vi "Setscope.vi"(10 "Set_Val":T1) -> (3 "OneOfTemplate out":refnum<class "nixnet_grpc_StartRequest_scope_enum.lvclass">)   [LabVIEW 2019, in "xnet-grpc_client.lvlib" / "nixnet_grpc_StartRequest_scope_enum.lvclass"]
uses:
  nixnet_grpc_StartRequest_scope_enum.lvclass
  nixnet_grpc_StartRequest_scope_enum.lvclass/nixnet_grpc_StartRequest_scope_enum.ctl
  nixnet_grpc_StartStopScope.ctl
  xnet-grpc_client.lvlib
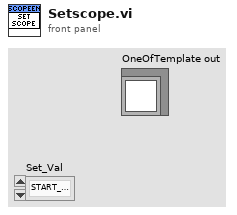
[diagram p1: front panel]
types:
  T1 = typedef "xnet-grpc_client.lvlib/nixnet_grpc_StartStopScope.ctl" = enum32{"START_STOP_SCOPE_NORMAL", "START_STOP_SCOPE_SESSION_ONLY", "START_STOP_SCOPE_INTERFACE_ONLY", "START_STOP_SCOPE_SESSION_ONLY_BLOCKING"}
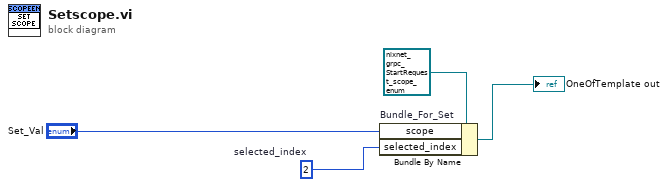
[diagram p0: block diagram]
diagram:
  w2 = 2  # selected_index
  n1 = Bundle By Name "Bundle_For_Set"(cluster=refnum<class "nixnet_grpc_StartRequest_scope_enum.lvclass"> refnum ("OneOfTemplate in"), "scope"="Set_Val", "selected_index"=w2) -> (→"OneOfTemplate out":refnum<class "nixnet_grpc_StartRequest_scope_enum.lvclass">)
